vi "13-type_digital_bis.vi"(3 "this":i32, 4 "Count in":i32, 5 "button":i32, 6 "Cluster":T1={"Auto1"=TRUE, "Auto2"=TRUE, "Rel1"=FALSE, "Rel2"=FALSE, "Filt1"=FALSE, "Filt2"=FALSE, "Rate"=enum."Slow", "Range1"=enum."10mV", "Range2"=enum."100mV", "Filt3"=FALSE, "Filt4"=FALSE, "Rel temp 1"=FALSE, "Analog1"=FALSE, "Analog2"=FALSE, "Analog temp 1"=FALSE, "Digital1"=FALSE, "Digital2"=FALSE, "Digital temp 1 "=FALSE, "Window1"=enum."None", "Window2"=enum."None", "Window temp 1"=enum."None", "RDGS1"="010", "RDGS2"="010", "RDGS temp 1"="010", "Type_type1"=TRUE, "Type_type2"=TRUE, "Type_type temp 1"=TRUE, "LSync"=FALSE, "Unit"=enum."C", "Sens"=TRUE, "Type tcoupl"=enum."J", "Junc"=TRUE, "prevState"=0, "Rel temp 2"=FALSE, "Analog temp 2"=FALSE, "Digital temp 2"=FALSE, "Type_type temp 2"=TRUE, "RDGS temp 2"="010", "Window temp 2"=enum."None", "address"="0", "digits"=0}) -> (0 "next state":i32, 1 "Count out":i32, 2 "Cluster 2":T1)   [LabVIEW 2017]
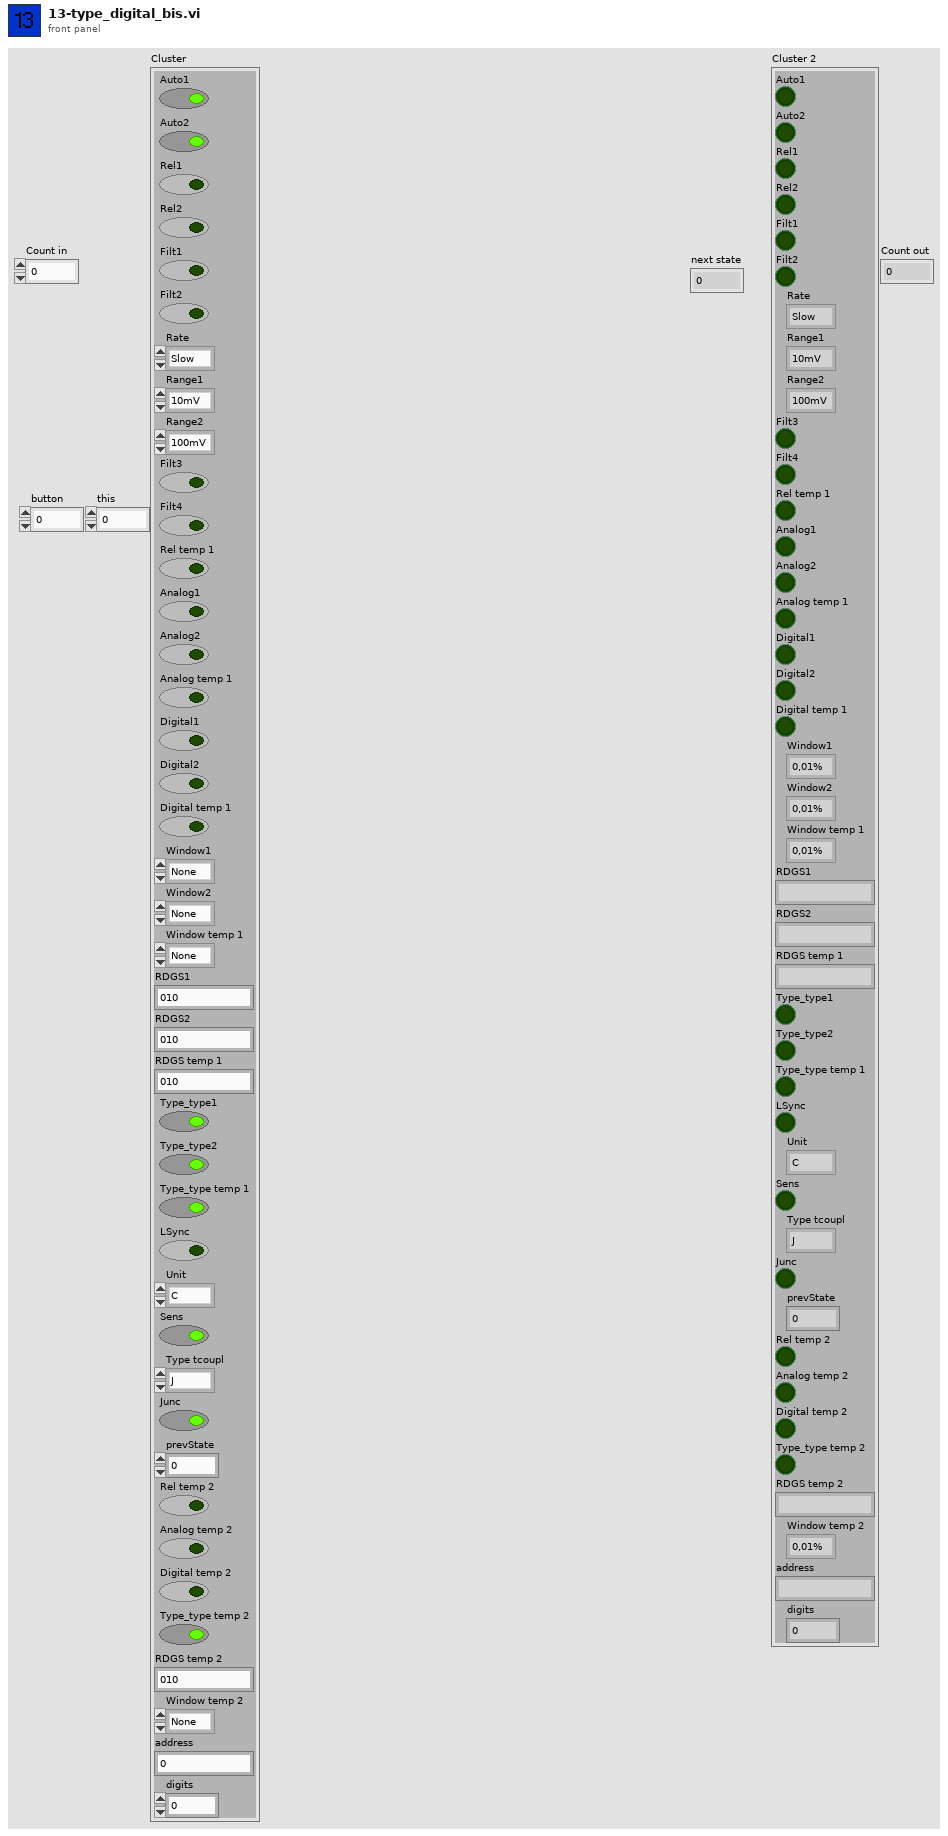
[diagram p1: front panel]
types:
  T1 = cluster{"Auto1":bool, "Auto2":bool, "Rel1":bool, "Rel2":bool, "Filt1":bool, "Filt2":bool, "Rate":enum16{"Slow", "Fast", "Med"}, "Range1":enum16{"10mV", "100mV", "1V", "10V", "100V"}, "Range2":enum16{"100mV", "1V", "10V"}, "Filt3":bool, "Filt4":bool, "Rel temp 1":bool, "Analog1":bool, "Analog2":bool, "Analog temp 1":bool, "Digital1":bool, "Digital2":bool, "Digital temp 1 ":bool, "Window1":enum16{"0,01%", "0,1%", "1%", "10%", "None"}, "Window2":enum16{"0,01%", "0,1%", "1%", "10%", "None"}, "Window temp 1":enum16{"0,01%", "0,1%", "1%", "10%", "None"}, "RDGS1":string, "RDGS2":string, "RDGS temp 1":string, "Type_type1":bool, "Type_type2":bool, "Type_type temp 1":bool, "LSync":bool, "Unit":enum16{"C", "K", "F"}, "Sens":bool, "Type tcoupl":enum16{"J", "K", "T", "E", "R", "S", "B", "N"}, "Junc":bool, "prevState":i32, "Rel temp 2":bool, "Analog temp 2":bool, "Digital temp 2":bool, "Type_type temp 2":bool, "RDGS temp 2":string, "Window temp 2":enum16{"0,01%", "0,1%", "1%", "10%", "None"}, "address":string, "digits":i32}
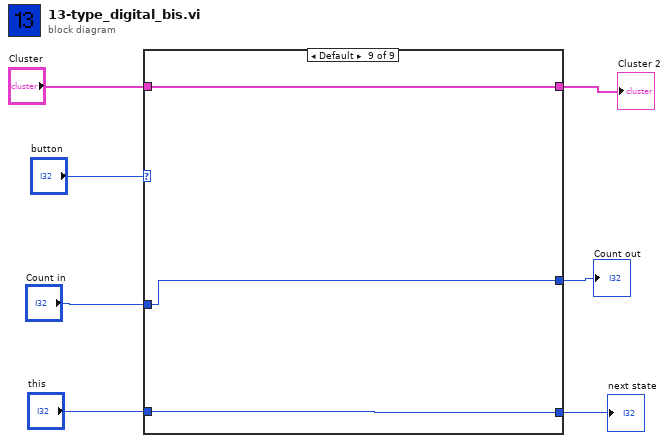
[diagram p0: block diagram]
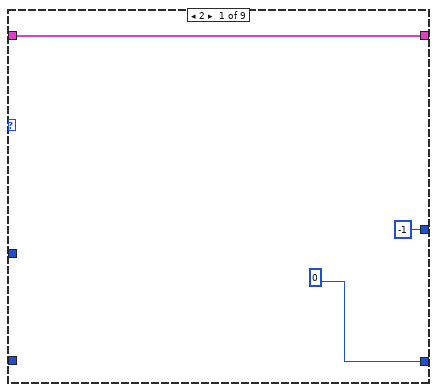
[diagram p2: hidden frame]
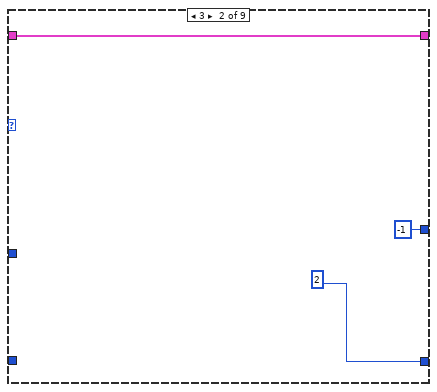
[diagram p3: hidden frame]
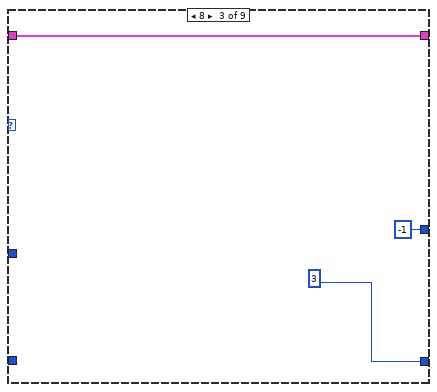
[diagram p4: hidden frame]
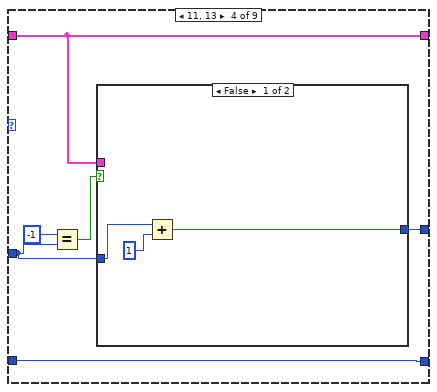
[diagram p5: hidden frame]
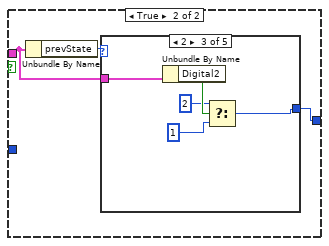
[diagram p6: hidden frame]
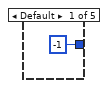
[diagram p7: hidden frame]
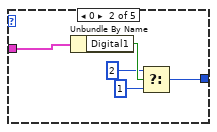
[diagram p8: hidden frame]
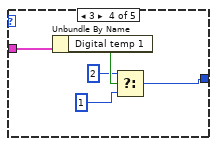
[diagram p9: hidden frame]
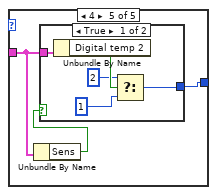
[diagram p10: hidden frame]
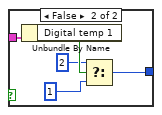
[diagram p11: hidden frame]
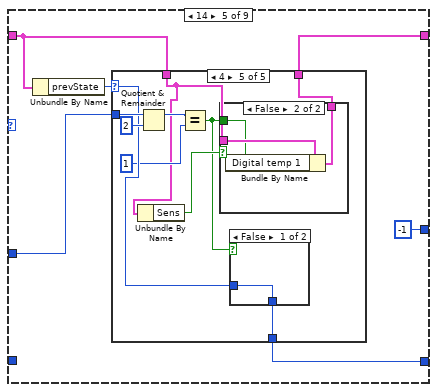
[diagram p12: hidden frame]
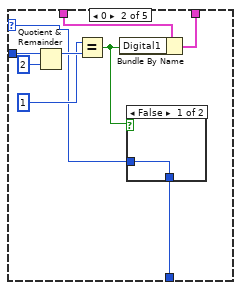
[diagram p14: hidden frame]
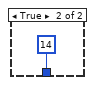
[diagram p15: hidden frame]
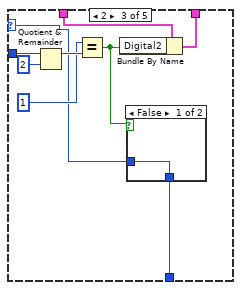
[diagram p16: hidden frame]
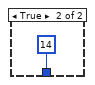
[diagram p17: hidden frame]
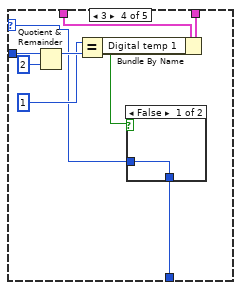
[diagram p18: hidden frame]
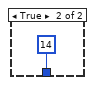
[diagram p19: hidden frame]
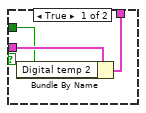
[diagram p20: hidden frame]
diagram:
  n1 = case shown="Default" "button" {
    tunnel: [0 ("this") 2 3 w18 w58 12 ("this") 4 w124 w127] -> w5
    tunnel: "this" -> [_ _ _ w18 _ _ _ _ w127]
    tunnel: "Cluster" -> [w10 w12 w15 w21 w63 w119 w121 w125 w128]
    tunnel: [w10 w12 w15 w21 w60 w119 w121 w125 w128] -> w4
    tunnel: "Count in" -> [_ _ _ w20 w59 _ _ _ w126]
    tunnel: [-1 ("t") -1 ("t") -1 ("t") w19 -1 ("t") -1 ("t") -1 ("t") -1 ("t") w126] -> w2
    frame 2 {
    }
    frame 3 {
    }
    frame 8 {
    }
    frame 11, 13 {
      n2 = Equal?(x=-1, y=w20) -> (x = y?=w22:bool)
      n3 = case shown="False" w22 {
        tunnel: w21 -> [_ w27]
        tunnel: w20 -> [w25 _]
        tunnel: [w23 w26] -> w19
        frame False {
          n4 = Add(x=w25, y=1) -> (x+y=w23:i32)
        }
        frame True {
          n5 = Unbundle By Name(w27) -> ("prevState"=w28:i32)
          n6 = case shown="2" w28 {
            tunnel: w27 -> [_ w34 w39 w44 w46]
            tunnel: [-1 ("t") w30 w35 w40 w47] -> w26
            frame Default {
            }
            frame 0 {
              n7 = Unbundle By Name(w34) -> ("Digital1"=w33:bool)
              n8 = Select(t=2, s=w33, f=1) -> (s? t:f=w30:i32)
            }
            frame 2 {
              n9 = Unbundle By Name(w39) -> ("Digital2"=w38:bool)
              n10 = Select(t=2, s=w38, f=1) -> (s? t:f=w35:i32)
            }
            frame 3 {
              n11 = Unbundle By Name(w44) -> ("Digital temp 1"=w43:bool)
              n12 = Select(t=2, s=w43, f=1) -> (s? t:f=w40:i32)
            }
            frame 4 {
              n13 = Unbundle By Name(w46) -> ("Sens"=w45:bool)
              n14 = case shown="True" w45 {
                tunnel: w46 -> [w52 w57]
                tunnel: [w48 w53] -> w47
                frame True {
                  n15 = Unbundle By Name(w52) -> ("Digital temp 2"=w51:bool)
                  n16 = Select(t=2, s=w51, f=1) -> (s? t:f=w48:i32)
                }
                frame False {
                  n17 = Unbundle By Name(w57) -> ("Digital temp 1"=w56:bool)
                  n18 = Select(t=2, s=w56, f=1) -> (s? t:f=w53:i32)
                }
              }
            }
          }
        }
      }
    }
    frame 14 {
      n19 = Unbundle By Name(w63) -> ("prevState"=w62:i32)
      n20 = case shown="4" w62 {
        selector: w62 -> [w65 w66 w77 w88 w105]
        tunnel: w63 -> [w64 w74 w85 w96 w101]
        tunnel: [w64 w73 w84 w95 w100] -> w60
        tunnel: w59 -> [_ w72 w83 w94 w108]
        tunnel: [w65 w67 w78 w89 w106] -> w58
        frame Default {
        }
        frame 0 {
          n21 = Quotient & Remainder(x=w72, y=2) -> (x-y*floor(x/y)=w70:i32)  [unwired: 1 out]
          n22 = Equal?(x=1, y=w70) -> (x = y?=w68:bool)
          n23 = Bundle By Name(cluster=w74, "Digital1"=w68) -> (w73:T1)
          n24 = case shown="False" w68 {
            tunnel: [w75 14] -> w67
            tunnel: w66 -> [w75 _]
            frame False {
            }
            frame True {
            }
          }
        }
        frame 2 {
          n25 = Quotient & Remainder(x=w83, y=2) -> (x-y*floor(x/y)=w81:i32)  [unwired: 1 out]
          n26 = Equal?(x=1, y=w81) -> (x = y?=w79:bool)
          n27 = Bundle By Name(cluster=w85, "Digital2"=w79) -> (w84:T1)
          n28 = case shown="False" w79 {
            tunnel: [w86 14] -> w78
            tunnel: w77 -> [w86 _]
            frame False {
            }
            frame True {
            }
          }
        }
        frame 3 {
          n29 = Quotient & Remainder(x=w94, y=2) -> (x-y*floor(x/y)=w92:i32)  [unwired: 1 out]
          n30 = Equal?(x=1, y=w92) -> (x = y?=w90:bool)
          n31 = Bundle By Name(cluster=w96, "Digital temp 1"=w90) -> (w95:T1)
          n32 = case shown="False" w90 {
            tunnel: [w97 14] -> w89
            tunnel: w88 -> [w97 _]
            frame False {
            }
            frame True {
            }
          }
        }
        frame 4 {
          n33 = Unbundle By Name(w101) -> ("Sens"=w104:bool)
          n34 = Quotient & Remainder(x=w108, y=2) -> (x-y*floor(x/y)=w103:i32)  [unwired: 1 out]
          n35 = Equal?(x=w103, y=1 ("x")) -> (x = y?=w99:bool)
          n36 = case shown="False" w104 {
            tunnel: w99 -> [w110 w113]
            tunnel: w101 -> [w111 w114]
            tunnel: [w109 w112] -> w100
            frame True {
              n37 = Bundle By Name(cluster=w111, "Digital temp 2"=w110) -> (w109:T1)
            }
            frame False {
              n38 = Bundle By Name(cluster=w114, "Digital temp 1"=w113) -> (w112:T1)
            }
          }
          n39 = case shown="False" w99 {
            tunnel: [w115 14] -> w106
            tunnel: w105 -> [w115 _]
            frame False {
            }
            frame True {
            }
          }
        }
      }
    }
    frame 15, 24 {
    }
    frame 16 {
    }
    frame 32 {
      n40 = Unbundle By Name(w125) -> ("prevState"=w124:i32)
    }
    frame Default {
    }
  }
  "next state" <- w5
  "Count out" <- w2
  "Cluster 2" <- w4
